vi "INI Properties Functional Variable_DStr-Scope SP.vi"(1 "Mode(Get)":T2=enum."Get", 7 "proper":T1) -> (8 "proper":T1)   [LabVIEW 2012]
uses:
  Function Variable Parameter Operations-Scope SP.ctl
  INI Properties_DStr-Scope SP.ctl
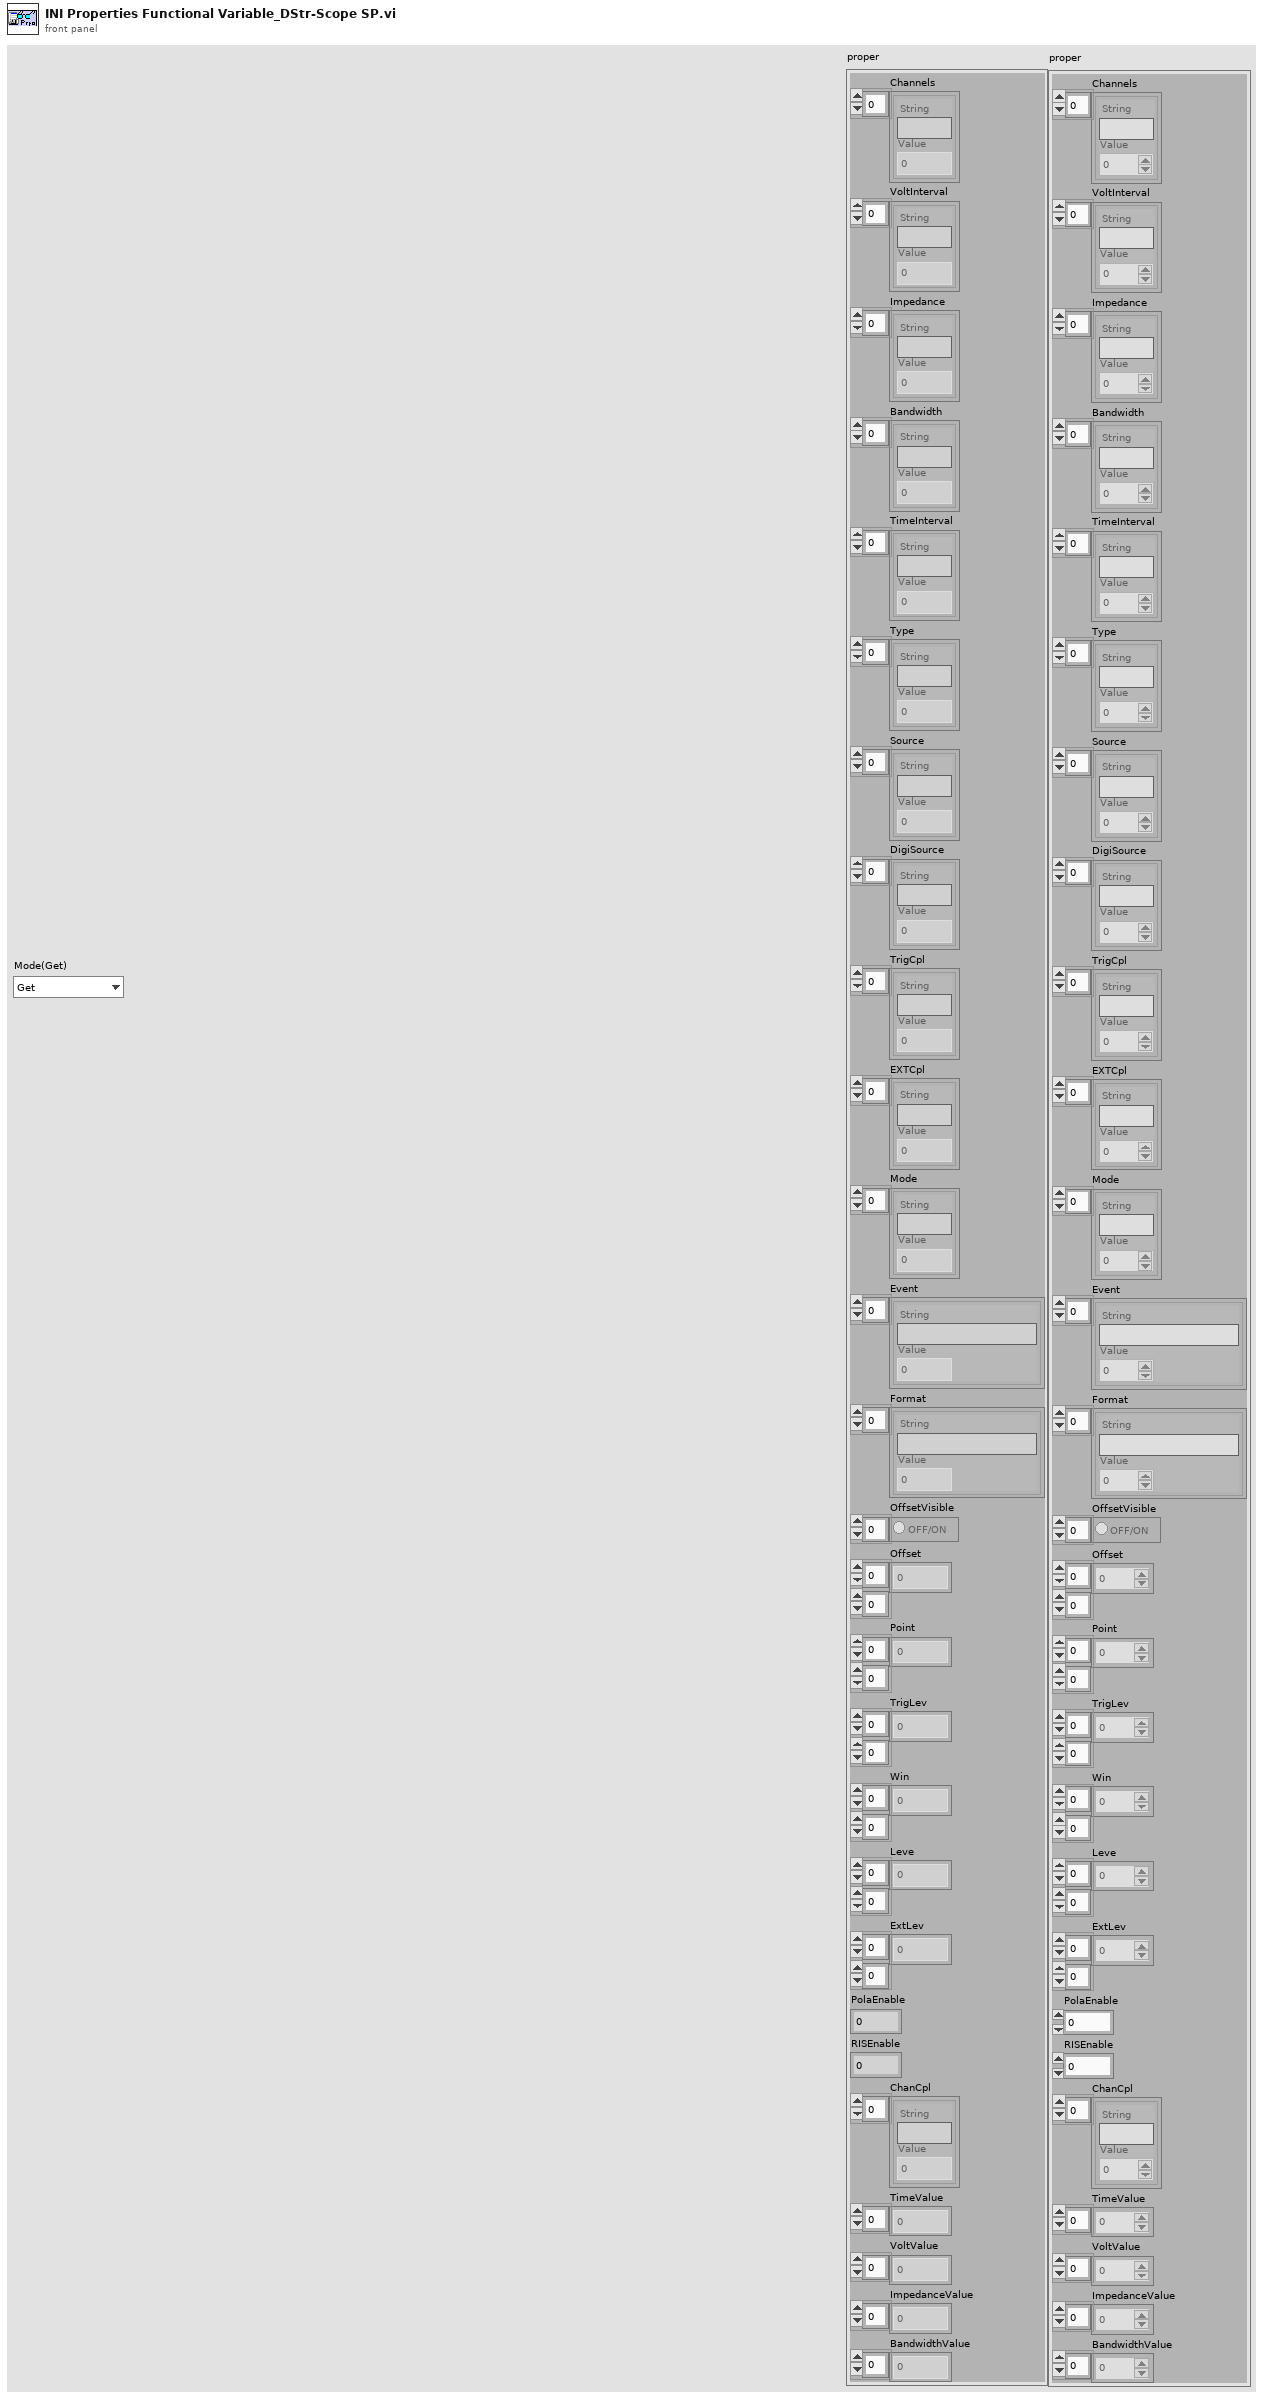
[diagram p1: front panel]
types:
  T1 = typedef "INI Properties_DStr-Scope SP.ctl" = cluster{"Channels":cluster{"String":string, "Value":ext}[], "VoltInterval":cluster{"String":string, "Value":ext}[], "Impedance":cluster{"String":string, "Value":ext}[], "Bandwidth":cluster{"String":string, "Value":ext}[], "TimeInterval":cluster{"String":string, "Value":ext}[], "Type":cluster{"String":string, "Value":ext}[], "Source":cluster{"String":string, "Value":ext}[], "DigiSource":cluster{"String":string, "Value":ext}[], "TrigCpl":cluster{"String":string, "Value":ext}[], "EXTCpl":cluster{"String":string, "Value":ext}[], "Mode":cluster{"String":string, "Value":ext}[], "Event":cluster{"String":string, "Value":ext}[], "Format":cluster{"String":string, "Value":ext}[], "OffsetVisible":bool[], "Offset":dbl[][], "Point":dbl[][], "TrigLev":dbl[][], "Win":dbl[][], "Leve":dbl[][], "ExtLev":dbl[][], "PolaEnable":u8, "RISEnable":u8, "ChanCpl":cluster{"String":string, "Value":ext}[], "TimeValue":dbl[], "VoltValue":dbl[], "ImpedanceValue":dbl[], "BandwidthValue":dbl[]}
  T2 = typedef "Function Variable Parameter Operations-Scope SP.ctl" = enum16{"Set", "Get"}
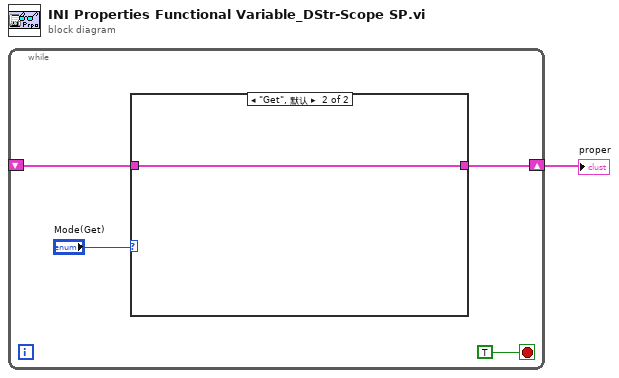
[diagram p0: block diagram]
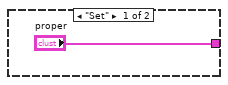
[diagram p2: hidden frame]
diagram:
  n1 = while {
    shift-right: [w3] -> w1
    shift-left: _ -> [w2]
    stop <- TRUE stop-if-true
    n2 = case shown="\"Get\", 默认" "Mode(Get)" {
      tunnel: ["proper" w7] -> w3
      tunnel: w2 -> [_ w7]
      frame "Set" {
      }
      frame "Get", Default {
      }
    }
  }
  "proper" <- w1
